vi "LOTTERY[1].vi"   [LabVIEW 2025]
uses:
  <vilib>/Utility/file.llb/Write Delimited Spreadsheet (DBL).vi
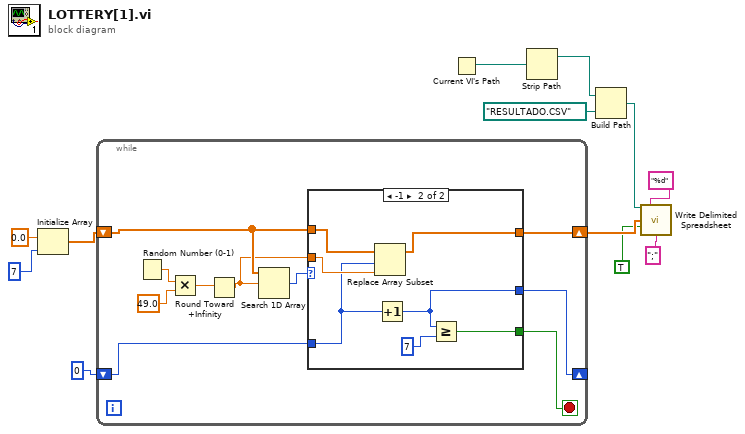
[diagram p0: block diagram]
diagram:
  n1 = Initialize Array(0.0 ("element"), 7) -> (w10:dbl[])
  n2 = while {
    shift-right: [w15] -> w2
    shift-left: w10 -> [w17]
    shift-right: [w14] -> _
    shift-left: 0 -> [w18]
    stop <- w13 stop-if-true
    n3 = Random Number (0-1)() -> (number: 0 to 1=w22:dbl)
    n4 = Multiply(x=w22, y=49.0) -> (x*y=w20:dbl)
    n5 = Round Toward +Infinity(x=w20) -> (ceil(x): smallest int >= x=w16:dbl)
    n6 = Search 1D Array(1D array=w17, element=w16) -> (index of element=w19:i32)  [unwired: 1 in]
    n7 = case shown="-1" w19 {
      tunnel: w18 -> [_ w26]
      tunnel: w17 -> [_ w29]
      tunnel: w16 -> [_ w28]
      tunnel: [_ w27] -> w15
      tunnel: [_ w25] -> w14
      tunnel: [_ w23] -> w13
      frame 0, Default {
      }
      frame -1 {
        n8 = Replace Array Subset(array=w29, new element=w28, index=w26) -> (w27:dbl[])
        n9 = Increment(x=w26) -> (x+1=w25:i32)
        n10 = Greater Or Equal?(x=w25, y=7) -> (x >= y?=w23:bool)
      }
    }
  }
  n11 = Current VI's Path() -> (path=w4:path)
  n12 = Strip Path(path=w4) -> (stripped path=w5:path)  [unwired: 1 out]
  n13 = Build Path(base path=w5, name or relative path=path "RESULTADO.CSV") -> (appended path=w6:path)
  n14 = call-poly <vilib>:"Write Delimited Spreadsheet.vi"("file path (dialog if empty)"=w6, "format (%.3f)"="%d", "1D data"=w2, "append to file? (new file:F)"=TRUE ("transpose? (no:F)"), "delimiter (\\t)"=";") -> ()  [unwired: 9 in, 2 out]
